vi "OAT Auto Window.vi"(6 "window info in":T1={"window type"=10, "window length"=2} {"window type" items=["None"=0, "Hanning"=1, "Hamming"=2, "Blackman-Harris"=3, "Exact Blackman"=4, "Blackman"=5, "Flat Top"=6, "4 Term B-Harris"=7, "7 Term B-Harris"=8, "Low Sidelobe"=9, "Gaussian"=62]; "window length" min=0}, 8 "error in (no error)":errorcluster, 10 "speed profile":T2 {"speed [RPM]" format="%.2f"; "time [s]" format="%.2f"}, 11 "scaled signal [EU]":waveform(dbl)={"t0"=timestamp(0 s since 1904-01-01), "dt"=0.0, "Y"=[]}) -> (0 "error out":errorcluster, 2 "speed profile out":T2 {"speed [RPM]" format="%.2f"; "time [s]" format="%.2f"}, 3 "scaled signal [EU] out":waveform(dbl), 4 "window info out":T1={"window type"=10, "window length"=2048} {"window type" items=["None"=0, "Hanning"=1, "Hamming"=2, "Blackman-Harris"=3, "Exact Blackman"=4, "Blackman"=5, "Flat Top"=6, "4 Term B-Harris"=7, "7 Term B-Harris"=8, "Low Sidelobe"=9, "Gaussian"=62]; "window length" min=0})   [LabVIEW 2017]
uses:
  <vilib>/addons/Sound and Vibration/Order Analysis/Tach Process/SubVIs/speed profile.ctl
  <vilib>/addons/Sound and Vibration/Order Analysis/Ref Gabor Order Tracking/window information.ctl
  <vilib>/Analysis/baseanly.llb/Mean (DBL).vi
  <vilib>/Analysis/NI_AALBase.lvlib
  <vilib>/addons/Sound and Vibration/Order Analysis/Tach Process/SoundVib_TachProcess.lvlib
  <vilib>/addons/Sound and Vibration/Order Analysis/Gabor Order Tracking/SoundVib_Gabor.lvlib
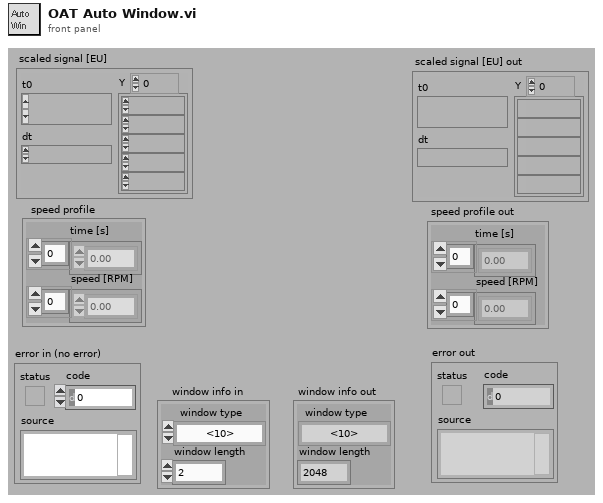
[diagram p1: front panel]
types:
  T1 = typedef "SoundVib_Gabor.lvlib/window information.ctl" = cluster{"window type":u32, "window length":i32}
  T2 = typedef "SoundVib_TachProcess.lvlib/speed profile.ctl" = cluster{"time [s]":dbl[], "speed [RPM]":dbl[]}
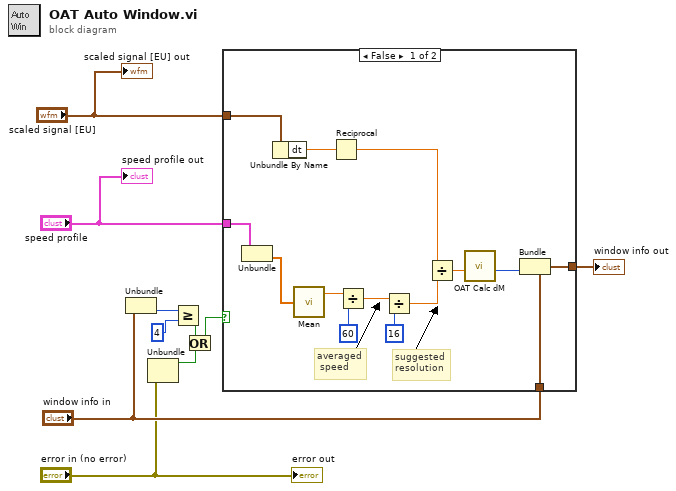
[diagram p0: block diagram]
diagram:
  n1 = Unbundle("window info in") -> ("window length"=w6:i32)  [unwired: 1 out]
  n2 = Unbundle("error in (no error)") -> ("status"=w3:bool)  [unwired: 2 out]
  n3 = Greater Or Equal?(x=w6, y=4) -> (x >= y?=w2:bool)
  n4 = Or(x=w2, y=w3) -> (x .or. y?=w1:bool)
  n5 = case shown="False" w1 {
    tunnel: "speed profile" -> [w24 _]
    tunnel: [w16 w25] -> w9
    tunnel: "scaled signal [EU]" -> [w15 _]
    tunnel: "window info in" -> [w11 w25]
    frame False {
      # "suggested\nresolution"
      # "averaged\n speed"
      n6 = Unbundle(w24) -> ("speed [RPM]"=w14:dbl[])  [unwired: 1 out]
      n7 = Unbundle By Name(w15) -> ("dt"=w19:dbl)
      n8 = call-poly <vilib>:"Mean.vi"("X"=w14) -> ("mean"=w23:dbl)  [unwired: 1 out]
      n9 = Reciprocal(x=w19) -> (1/x=w17:dbl)
      n10 = Divide(x=w23, y=60) -> (x/y=w21:dbl)
      n11 = Divide(x=w21, y=16) -> (x/y=w18:dbl)
      n12 = Divide(x=w17, y=w18) -> (x/y=w13:dbl)
      n13 = call <vilib>:"OAT Calc dM.vi"("window length"=w13) -> ("actual window length"=w12:i32)  [unwired: 7 in, 3 out]
      n14 = Bundle(cluster=w11, "window length"=w12) -> (w16:T1)  [unwired: 1 in]
    }
    frame True {
    }
  }
  "window info out" <- w9
  "scaled signal [EU] out" <- "scaled signal [EU]"
  "speed profile out" <- "speed profile"
  "error out" <- "error in (no error)"
